vi "set up image stack aquisition.vi"(7 "inter-frame interval (ms)":dbl=200.0, 8 "error in (no error)":errorcluster, 9 "extension":string="jpg", 10 "Field Width (0 disables 0 padding)":u8, 11 "stub":string) -> (0 "error out":errorcluster, 1 "camera image is 8 bit":bool, 2 "camera image":T2, 3 "stack read info":T1={"file stub"="", "format string"="%00d.%s", "extension"="jpg", "inter-frame interval (ms)"=0.0})   [LabVIEW 2021]
uses:
  <vilib>/vision/Image Controls.llb/IMAQ Image.ctl
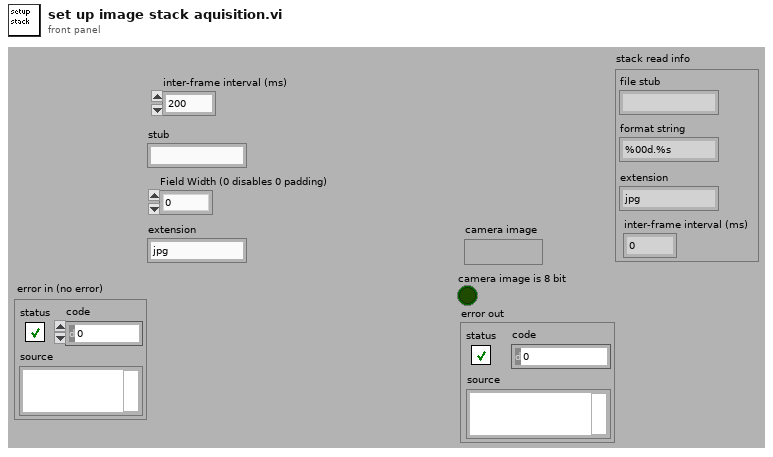
[diagram p1: front panel]
types:
  T1 = cluster{"file stub":string, "format string":string, "extension":string, "inter-frame interval (ms)":dbl}
  T2 = typedef "IMAQ Image.ctl" = refnum<image>
  T3 = typedef "Image Type" = u32
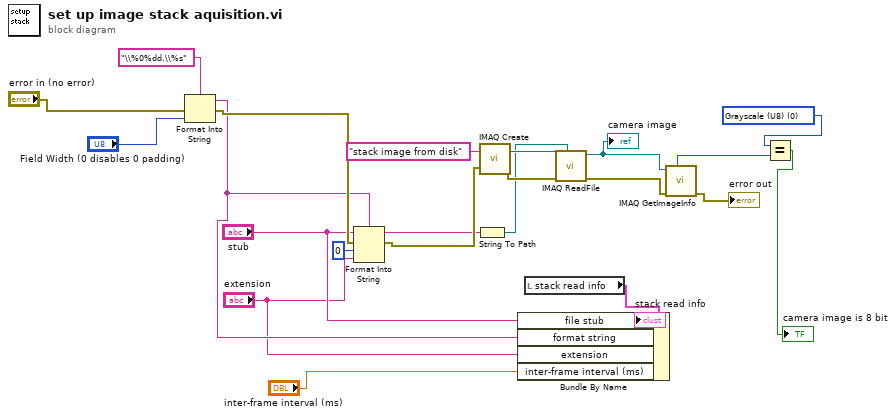
[diagram p0: block diagram]
diagram:
  w4 = T3 0 items=["Grayscale (U8)", "Grayscale (I16)", "Grayscale (SGL)", "Complex (CSG)", "RGB (U32)", "HSL (U32)", "RGB (U64)", "Grayscale (U16)"] ("Image Type")
  n1 = Format Into String(format string="\\%0%dd.\\%s", error in="error in (no error)", "Field Width (0 disables 0 padding)") -> (resulting string=w10:string, error out=w18:errorcluster)  [unwired: 1 in]
  n2 = Format Into String(format string=w10, initial string="stub", error in=w18, 0 ("input 1"), "extension") -> (resulting string=w15:string, error out=w17:errorcluster)
  n3 = String To Path(string=w15) -> (path=w14:path)
  n4 = call "IMAQ Create"("Image Name"="stack image from disk", "error in (no error)"=w17) -> ("New Image"=w20:T2, "error out"=w16:errorcluster)  [unwired: 3 in]
  n5 = local read "stack read info"() -> (w12:T1)
  n6 = Bundle By Name(cluster=w12, "file stub"="stub", "format string"=w10, "extension"="extension", "inter-frame interval (ms)"="inter-frame interval (ms)") -> (→"stack read info":T1)
  n7 = call "IMAQ ReadFile"("File Path"=w14, "error in (no error)"=w16, "Image"=w20) -> ("error out"=w6:errorcluster, "Image Out"=w5:T2)  [unwired: 4 in, 3 out]
  "camera image" <- w5
  n8 = call "IMAQ GetImageInfo"("error in (no error)"=w6, "Image"=w5) -> ("error out"=→"error out":errorcluster, "Image Type"=w3:T3)  [unwired: 2 in, 6 out]
  n9 = Equal?(x=w4, y=w3) -> (x = y?=→"camera image is 8 bit":bool)
